vi "Actor Core.vi"(8 "error in":errorcluster, 11 "Assert Service in":refnum<class "Assert Service.lvclass">) -> (0 "error out":errorcluster, 3 "Actor out":refnum<class "Actor.lvclass">)   [LabVIEW 2016, in "Assert API Components.lvlib" / "Assert Service.lvlib" / "Assert Service.lvclass"]
doc: "(<B>Filename</B>: Actor Framework.lvlib:Actor.lvclass:Actor Core.vi)\n\nReceives messages to the actor, reacts to them, and initiates any error handling that may shut the actor down.\n\nDescendant classes may override this VI to append parallel tasks for the actor to complete while it handles messages. Overrides use the Call Parent Method node."
uses:
  Assert Service.lvclass
  <vilib>/ActorFramework/Actor/Actor.lvclass
  D:/Work/Projects/actor_assert_api/Core/Base UI Actor/Base UI Actor/Base UI Actor.lvclass
  C:/Program Files (x86)/National Instruments/LabVIEW 2016/vi.lib/ActorFramework/Actor/Actor.lvclass
  Service States.ctl
  <vilib>/NI/STM/TCP/TCP Connection Info.ctl
  <vilib>/NI/STM/SubVIs/MetaDataElement.ctl
  <vilib>/ActorFramework/Actor/Actor.lvclass/Actor.ctl
  Base UI Actor/Base UI Actor/Base UI Actor.lvclass/Base UI Actor.ctl
  Assert Service.lvclass/Assert Service.ctl
  <vilib>/NI/STM/TCP/TCP Read Options.ctl
  <vilib>/NI/STM/TCP/Get Connection Reference (TCP).vi
  <vilib>/NI/STM/TCP/Read Message (TCP).vi
  Base UI Actor/Base UI Actor/Base UI Actor.lvclass
  <vilib>/NI/STM/NI STM.lvlib
  Assert Service.lvlib
panel:
  out "IP Address":string
  out "Service Name":string
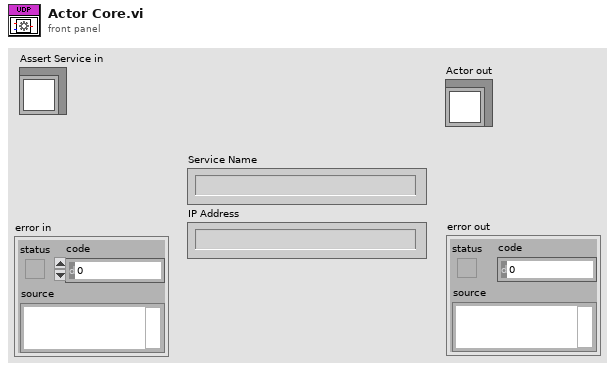
[diagram p1: front panel]
types:
  T1 = typedef "NI STM.lvlib/TCP Connection Info.ctl" = cluster{"connection ID":refnum<k5>, "meta data":T2[]}
  T2 = typedef "NI STM.lvlib/MetaDataElement.ctl" = string
  T3 = typedef "Assert API Components.lvlib/Assert Service.lvlib/Service States.ctl" = enum16{"Generate Link", "Acquire Data"}
  T4 = typedef "NI STM.lvlib/TCP Read Options.ctl" = cluster{"ignore timeout error":bool, "timeout ms (1000)":i32}
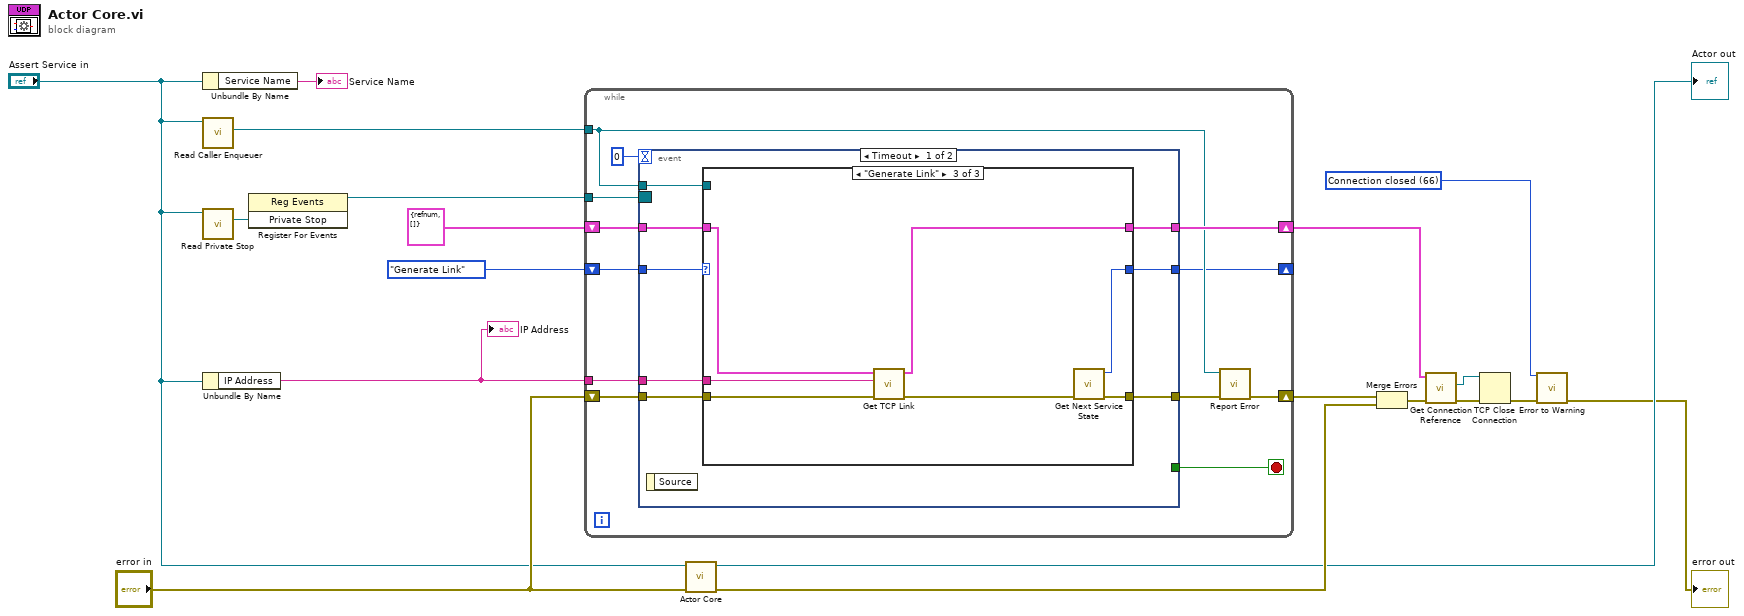
[diagram p0: block diagram]
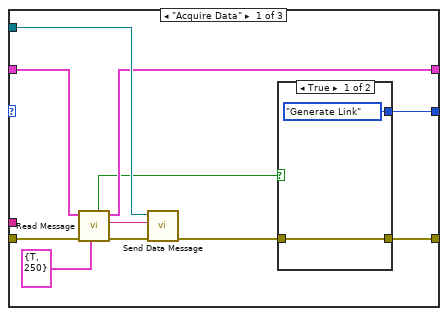
[diagram p2: hidden frame]
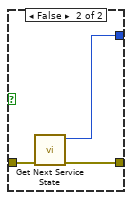
[diagram p3: hidden frame]
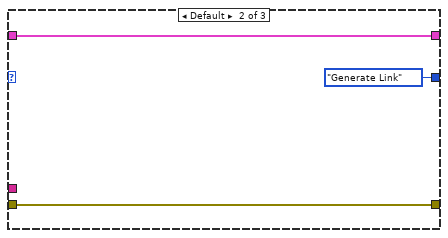
[diagram p4: hidden frame]
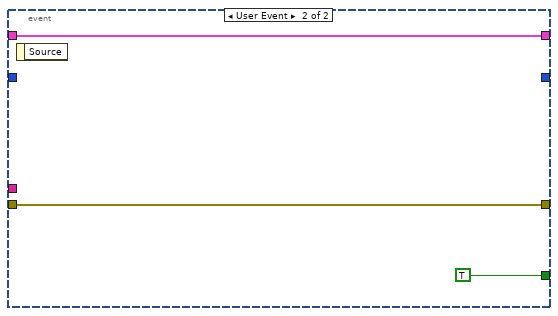
[diagram p5: hidden frame]
diagram:
  w10 = 66 items=["No Error", "Argument Error", "Memory Full", "Out of Zone", "End of File", "File Already Open", "Generic File IO Error", "File Not Found", "File Permission Error", "Disk Full", "Duplicate Path", "Too Many Files Open", "Not Enabled", "Resource File Not Found", "Cannot Add Resource", "Resource Not Found", "Image Not Found", "Image Memory Error", "Pen Does Not Exist", "Config Bad Type", "Config Token Not Found", "Config Parse Error", "Config Memory Error", "Bad External Code Format", "Bad External Code Offset", "External Code Not Present", "Null Window", "Destroy Window Mixup", "Null Menu", "Print Aborted", "Bad Print Record", "Print Driver Error", "Windows Error During Print", "Memory Error During Print", "Print Dialog Error", "Generic Print Error", "Invalid Device Refnum", "Device Not Found", "Device Parameter Error", "Device Unit Error", "Can't Open Device", "Device Call Aborted", "Generic Error", "Cancelled By User", "Object ID Too Low", "Object ID Too High", "Object Not In Heap", "Unknown Heap", "Bad DefProc ID", "DefProc Not In Table", "Message Out Of Range", "Null Method", "Unknown Message", "Manager Call Not Supported", "Bad address", "Connection In progress", "Connection timed out", "Connection is already in progress", "Network attribute not supported", "Network error", "Address in use", "System out of memory", "Connection aborted", "Connection refused", "Connection is not connected", "Connection is already connected", "Connection closed", "Initialize error (interapplication manager)", "Bad occurrence", "Wait on unbound occurrence handler", "Occurrence queue overflow", "Bad path", "Semaphore not signaled", "Unrecognized type (interapplication manager)"] ("1st Error to Convert")
  n1 = Unbundle By Name("Assert Service in") -> ("Service Name"=→"Service Name":string)
  n2 = call <vilib>:"Read Caller Enqueuer.vi"("Actor"="Assert Service in") -> ("Caller Enqueuer"=w14:refnum<class "Message Enqueuer.lvclass">)  [unwired: 10 in]
  n3 = call "Read Private Stop.vi"("Base UI Actor in"="Assert Service in") -> ("Private Stop"=w17:refnum<user-event>)  [unwired: 10 in]
  n4 = Unbundle By Name("Assert Service in") -> ("IP Address"=w1:string)
  "IP Address" <- w1
  n5 = register-events(w17) -> (reference out=w16:refnum<event-registration>)  [unwired: 2 in, 1 out]
  n6 = while {
    tunnel: w16 -> [w31]
    tunnel: w14 -> [w25]
    shift-right: [w26] -> w5
    shift-left: T1 {"connection ID"=refnum, "meta data"=[]} ("connection info out") -> [w28]
    shift-right: [w23] -> w13
    shift-left: "error in" -> [w27]
    tunnel: w1 -> [w22]
    shift-right: [w20] -> _
    shift-left: Service_States."Generate Link" -> [w21]
    stop <- w29 stop-if-true
    n7 = event shown="[0] Timeout" {
      selector: w31 -> [_ _]
      dyn-events: _ -> [_ _]
      timeout: 0 -> [_ _]
      tunnel: [_ TRUE] -> w29
      tunnel: w28 -> [w39 w67]
      tunnel: w27 -> [w38 w66]
      tunnel: w25 -> [w37 _]
      tunnel: [w36 w66] -> w24
      tunnel: [w35 w67] -> w26
      tunnel: w22 -> [w32 _]
      tunnel: w21 -> [w34 _]
      tunnel: [w33 _] -> w20
      event Timeout {
        n8 = event-data() -> ()  [unwired: 1 in, 1 out]
        n9 = case shown="\"Generate Link\"" w34 {
          tunnel: w39 -> [w48 w58 w60]
          tunnel: w38 -> [w47 w57 w65]
          tunnel: w37 -> [w46 _ _]
          tunnel: [w42 w57 w63] -> w36
          tunnel: [w44 w58 w61] -> w35
          tunnel: [w43 Service_States."Generate Link" w62] -> w33
          tunnel: w32 -> [_ _ w59]
          frame "Acquire Data" {
            n10 = call-poly <vilib>:"Read Message.vi"("options"=T4 {"ignore timeout error"=TRUE, "timeout ms (1000)"=250}, "error in"=w47, "connection info in"=w48) -> ("error out"=w49:errorcluster, "data string"=w50:string, "connection info out"=w44:T1, "timed out?"=w40:bool)  [unwired: 3 in, 2 out]
            n11 = call "Send Data Message.vi"("error in (no error)"=w49, "data string"=w50, "Message Enqueuer in"=w46) -> ("error out"=w41:errorcluster)  [unwired: 8 in]
            n12 = case shown="True" w40 {
              tunnel: [Service_States."Generate Link" ("Service States") w55] -> w43
              tunnel: [w51 w54] -> w42
              tunnel: w41 -> [w51 w53]
              frame True {
              }
              frame False {
                n13 = call "Get Next Service State.vi"("error in (no error)"=w53) -> ("error out"=w54:errorcluster, "Service States"=w55:T3)  [unwired: 9 in]
              }
            }
          }
          frame Default {
          }
          frame "Generate Link" {
            n14 = call "Get TCP Link.vi"("error in (no error)"=w65, "IP Address"=w59, "connection info in"=w60) -> ("error out"=w64:errorcluster, "connection info out"=w61:T1)  [unwired: 7 in]
            n15 = call "Get Next Service State.vi"("error in (no error)"=w64) -> ("error out"=w63:errorcluster, "Service States"=w62:T3)  [unwired: 9 in]
          }
        }
      }
      event User Event {
        n16 = event-data() -> ()  [unwired: 1 in, 1 out]
      }
    }
    n17 = call "Report Error.vi"("error in (no error)"=w24, "Self Enqueuer"=w25) -> ("error out"=w23:errorcluster)  [unwired: 9 in]
  }
  n18 = call-parent "Actor Core.vi"("error in"="error in", "Actor in"="Assert Service in") -> ("error out"=w19:errorcluster, "Actor out"=→"Actor out":refnum<class "Actor.lvclass">)  [unwired: 8 in]
  n19 = Merge Errors(w13, w19) -> (w7:errorcluster)
  n20 = call-poly <vilib>:"Get Connection Reference.vi"("error in"=w7, "connection info in"=w5) -> ("error out"=w9:errorcluster, "connection ID out"=w8:refnum<k5>)  [unwired: 8 out]
  n21 = TCP Close Connection(connection ID=w8, error in (no error)=w9) -> (error out=w11:errorcluster)  [unwired: 2 out]
  n22 = call <vilib>:"Error to Warning.vi"("1st Error to Convert"=w10, "error in"=w11) -> ("warning out"=→"error out":errorcluster)  [unwired: 3 in, 10 out]
